vi "Get BufferLastReadsDBL.lvclass.vi"(11 "Thermometer DAQmx TC Cont CFG in":refnum<class "Thermometer DAQmx TC Cont CFG.lvclass">) -> (2 "BufferLastReadsDBL.lvclass":refnum<class "BufferLastReadsDBL.lvclass">, 3 "Thermometer DAQmx TC Cont CFG out":refnum<class "Thermometer DAQmx TC Cont CFG.lvclass">)   [LabVIEW 2024, in "Thermometer DAQmx TC Cont CFG.lvclass"]
uses:
  Thermometer DAQmx TC Cont CFG.lvclass
  Thermometer DAQmx TC Cont CFG.lvclass/Thermometer DAQmx TC Cont CFG.ctl
  Buffers/BufferLastReadingsDBL/BufferLastReadsDBL.lvclass
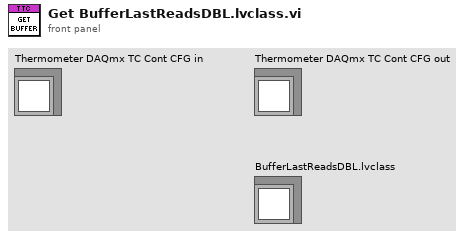
[diagram p1: front panel]
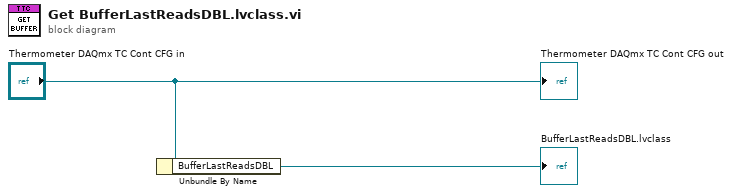
[diagram p0: block diagram]
diagram:
  n1 = Unbundle By Name("Thermometer DAQmx TC Cont CFG in") -> ("BufferLastReadsDBL"=→"BufferLastReadsDBL.lvclass":refnum<class "BufferLastReadsDBL.lvclass">)
  "Thermometer DAQmx TC Cont CFG out" <- "Thermometer DAQmx TC Cont CFG in"
